vi "RealCustomer.vi"(8 "error in (no error)":errorcluster, 10 "name":string, 11 "RealCustomer in":refnum<class "RealCustomer.lvclass">) -> (0 "error out":errorcluster, 3 "RealCustomer out":refnum<class "RealCustomer.lvclass">)   [LabVIEW 2017, in "RealCustomer.lvclass"]
uses:
  RealCustomer.lvclass
  RealCustomer.lvclass/RealCustomer.ctl
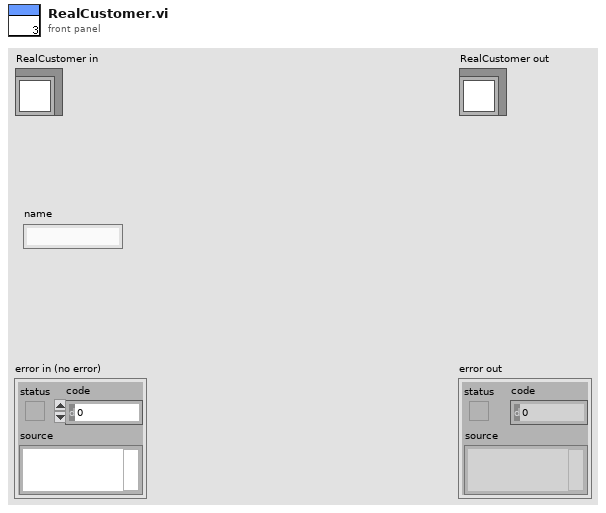
[diagram p1: front panel]
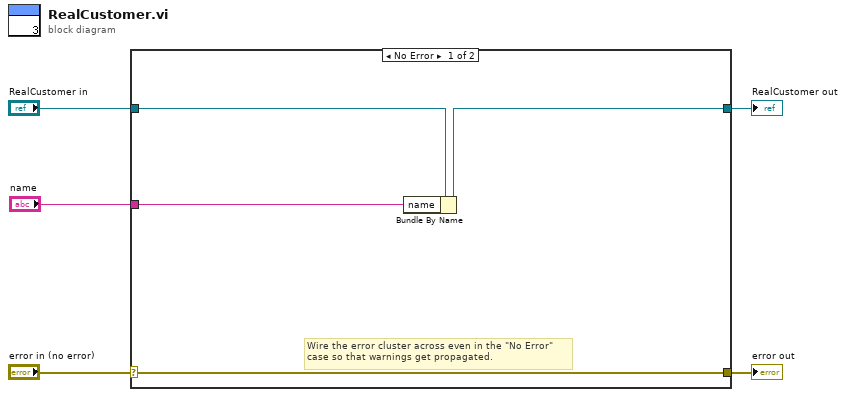
[diagram p0: block diagram]
diagram:
  n1 = case shown="No Error" "error in (no error)" {
    selector: "error in (no error)" -> [w8 w11]
    tunnel: [w8 w11] -> w4
    tunnel: [w7 w10] -> w2
    tunnel: "RealCustomer in" -> [w9 w10]
    tunnel: "name" -> [w6 _]
    frame No Error {
      # "Wire the error cluster across even in the \"No Error\"\ncase so that warnings get propagated."
      n2 = Bundle By Name(cluster=w9, "name"=w6) -> (w7:refnum<class "RealCustomer.lvclass">)
    }
    frame Error {
    }
  }
  "error out" <- w4
  "RealCustomer out" <- w2
